vi "ConvertCSVLogToPlots.vi"(11 "CSV String":string) -> (3 "Plots":cluster{timestamp[], "Y Data":dbl[]}[](array[cluster]))   [LabVIEW 2012]
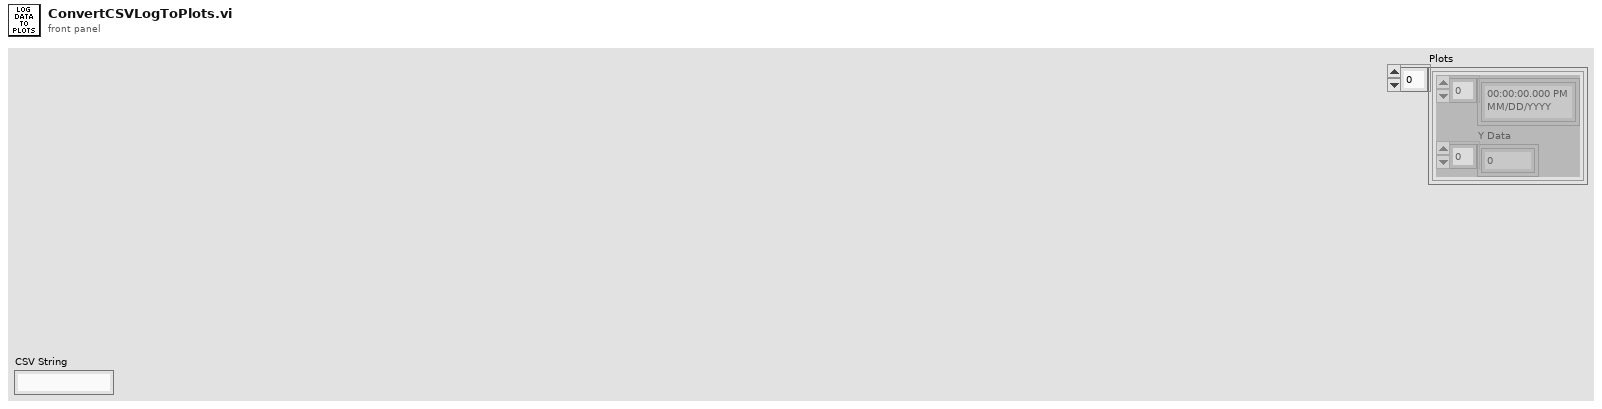
[diagram p1: front panel]
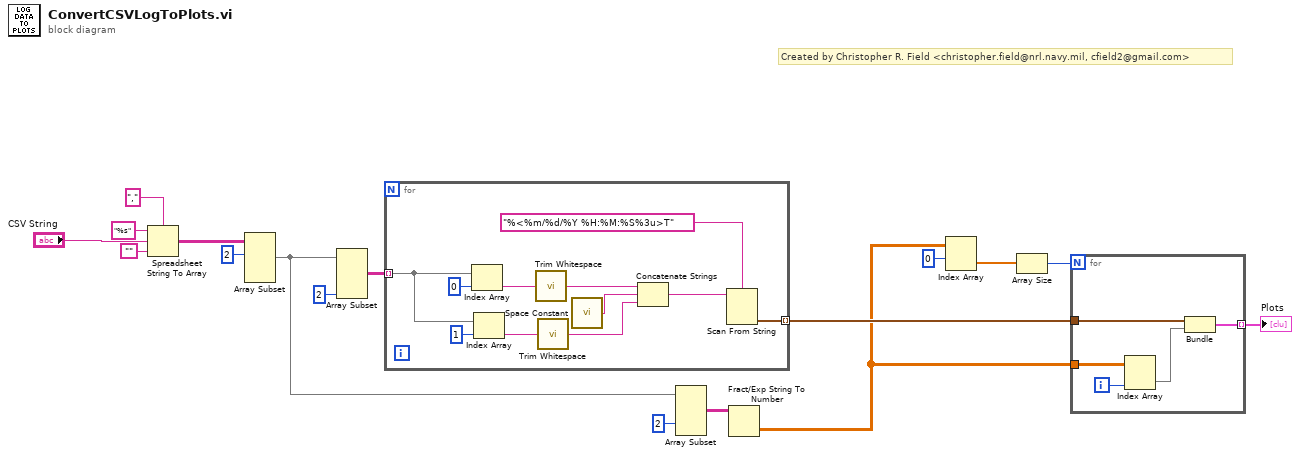
[diagram p0: block diagram]
diagram:
  # "Created by Christopher R. Field <christopher.field@nrl.navy.mil, cfield2@gmail.com>"
  n1 = Spreadsheet String To Array(delimiter (Tab)=",", format string="%s", spreadsheet string="CSV String", array type (2D Dbl)="") -> (array=w2:string[][])
  n2 = Array Subset(array=w2, index (row)=2 ("index")) -> (w6:string[][])  [unwired: 3 in]
  n3 = Array Subset(array=w6, length (col)=2 ("length")) -> (w13:string[][])  [unwired: 3 in]
  n4 = for {
    tunnel: w13 -> [w27] mode=indexing
    tunnel: [w18] -> w12 mode=indexing
    n5 = Index Array(array=w27, index=0) -> (element=w20:string)
    n6 = Index Array(array=w27, index=1) -> (element=w22:string)
    n7 = call <vilib>:"Trim Whitespace.vi"("string"=w20) -> ("trimmed string"=w19:string)  [unwired: 1 in]
    n8 = call <vilib>:"Trim Whitespace.vi"("string"=w22) -> ("trimmed string"=w21:string)  [unwired: 1 in]
    n9 = call <vilib>:"Space Constant.vi"() -> ("String"=w24:string)
    n10 = Concatenate Strings(w19, w24, w21) -> (w23:string)
    n11 = Scan From String(format string="%<%m/%d/%Y %H:%M:%S%3u>T", input string=w23) -> (output 1=w18:timestamp)  [unwired: 3 in, 3 out]
  }
  n12 = Array Subset(array=w6, index (col)=2 ("index")) -> (w10:string[][])  [unwired: 3 in]
  n13 = Fract/Exp String To Number(string=w10) -> (number=w8:dbl[][])  [unwired: 3 in, 1 out]
  n14 = Index Array(array=w8, index (row)=0) -> (element=w16:dbl[])  [unwired: 1 in]
  n15 = Array Size(array=w16) -> (size(s)=w15:i32)
  n16 = for {
    N: w15 -> [_]
    tunnel: w8 -> [w32]
    tunnel: [w33] -> w11 mode=indexing
    tunnel: w12 -> [w29]
    i -> [w31]
    n17 = Index Array(array=w32, index (col)=w31) -> (element=w30:dbl[])  [unwired: 1 in]
    n18 = Bundle(w29, w30) -> (w33:cluster{timestamp[], dbl[]})  [unwired: 1 in]
  }
  "Plots" <- w11
